vi "tearDown.vi"(8 "error in (no error)":errorcluster, 11 "reference in":refnum<class "labview-config-library.lvclass">) -> (0 "error out":errorcluster, 3 "reference out":refnum<class "labview-config-library.lvclass">)   [LabVIEW 2017, in "labview-config-library.lvclass"]
doc: "tearDown runs after the test method has completed. Use this method to clean up any operations or references that were opened by setUp or the test method. Unit tests should be independent of other unit tests so this VI should ensure that the next test can run in a 'clean' test environment."
uses:
  labview-config-library.lvclass
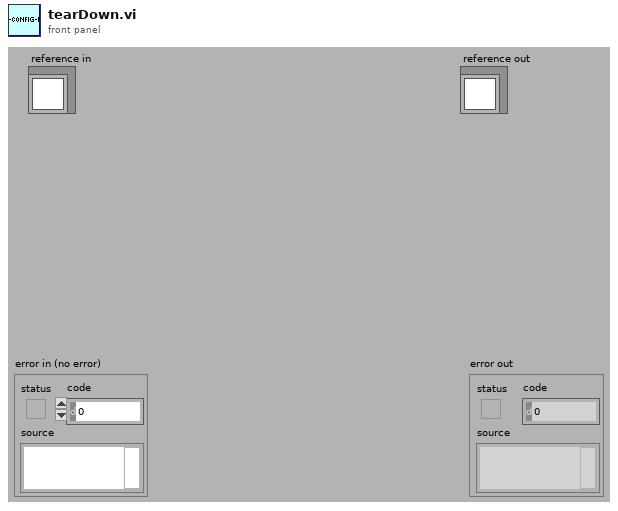
[diagram p1: front panel]
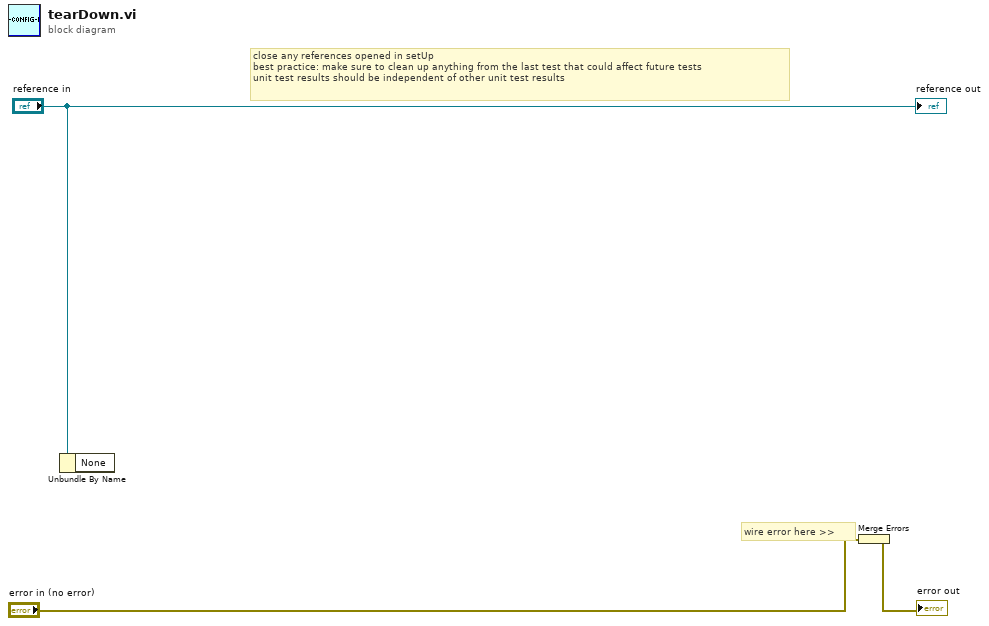
[diagram p0: block diagram]
diagram:
  # "wire error here >>"
  # "close any references opened in setUp\nbest practice: make sure to clean up anything from the last test that could affect future tests\nunit test results should be independent of other unit test results"
  n1 = Unbundle By Name("reference in") -> ()  [unwired: 1 out]
  n2 = Merge Errors("error in (no error)") -> (→"error out":errorcluster)
  "reference out" <- "reference in"
